vi "FTW-WebServer-Listener.vi"(1 "Endpoint":refnum<class "FTW-Endpoint.lvclass">, 2 "Message Handler":refnum<user-event>) -> ()   [LabVIEW 2015, in "FTW-WebServer.lvclass"]
uses:
  FTW-WebServer.lvclass
  Endpoint/FTW-Endpoint.lvclass
  Message/HttpRequest/FTW-Message-HttpRequest.lvclass
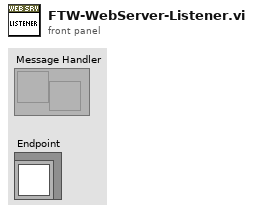
[diagram p1: front panel]
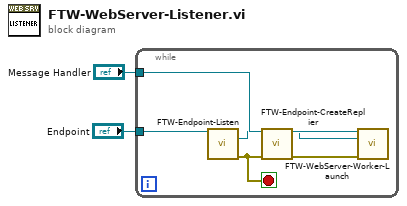
[diagram p0: block diagram]
diagram:
  n1 = while {
    tunnel: "Message Handler" -> [w7]
    tunnel: "Endpoint" -> [w8]
    stop <- w5 stop-if-true
    n2 = call-dynamic "FTW-Endpoint-Listen.vi"("FTW Endpoint"=w8) -> ("New Connection"=w6:refnum<class "FTW-Endpoint.lvclass">, "error out"=w5:errorcluster)  [unwired: 12 in, 1 out]
    n3 = call-dynamic "FTW-Endpoint-CreateReplier.vi"("FTW-Endpoint In"=w6, "error in"=w5) -> ("FTW-Endpoint Out"=w4:refnum<class "FTW-Endpoint.lvclass">, "error out"=w3:errorcluster)  [unwired: 12 in]
    n4 = call "FTW-WebServer-Worker-Launch.vi"("Message Handler"=w7, "FTW-Endpoint in"=w4, "error in"=w3) -> ()  [unwired: 12 in, 1 out]
  }
